vi "Supply_Init.vi"(8 "error in (no error)":errorcluster, 11 "SupplyControl in":refnum<class "SupplyControl.lvclass">) -> (0 "error out":errorcluster, 3 "SupplyControl out":refnum<class "SupplyControl.lvclass">)   [LabVIEW 2013, in "SupplyControl.lvclass"]
uses:
  SupplyControl.lvclass
  InstrControl.lvclass
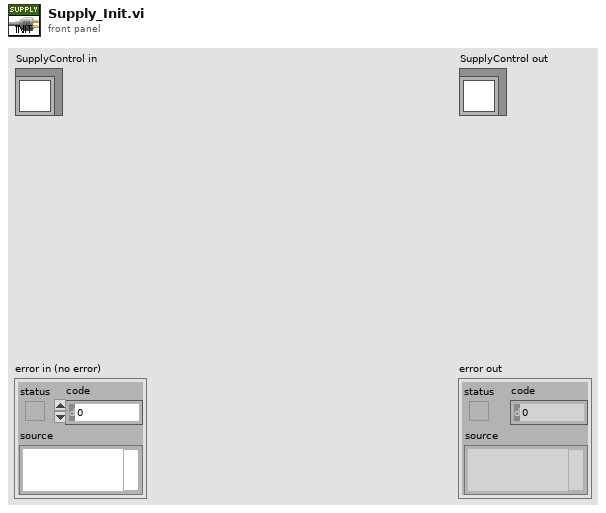
[diagram p1: front panel]
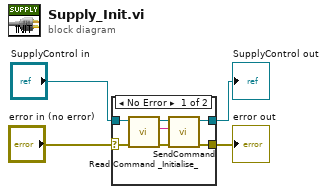
[diagram p0: block diagram]
diagram:
  n1 = case shown="No Error" "error in (no error)" {
    selector: "error in (no error)" -> [w10 w13]
    tunnel: [w9 w13] -> w3
    tunnel: [w5 w12] -> w1
    tunnel: "SupplyControl in" -> [w11 w12]
    frame No Error {
      n2 = call-dynamic "Read Command _Initialise_.vi"("error in (no error)"=w10, "SupplyControl in"=w11) -> ("error out"=w8:errorcluster, "Command \"Initialise\""=w7:string, "SupplyControl out"=w6:refnum<class "SupplyControl.lvclass">)  [unwired: 7 in]
      n3 = call "SendCommand.vi"("error in (no error)"=w8, "Command string"=w7, "InstControl in"=w6) -> ("error out"=w9:errorcluster, "InstControl out"=w5:refnum<class "SupplyControl.lvclass">)  [unwired: 7 in]
    }
    frame Error {
    }
  }
  "error out" <- w3
  "SupplyControl out" <- w1
